vi "Conveyor_SendToServer.vi"(6 "Cluster":T1, 7 "Emergency":bool, 8 "State":string, 9 "RPM in":dbl(knob) scale=0.0..10.0, 10 "Speed in":i32(listbox), 11 "Temperature in":dbl(slide) scale=0.0..100.0) -> ()   [LabVIEW 2026]
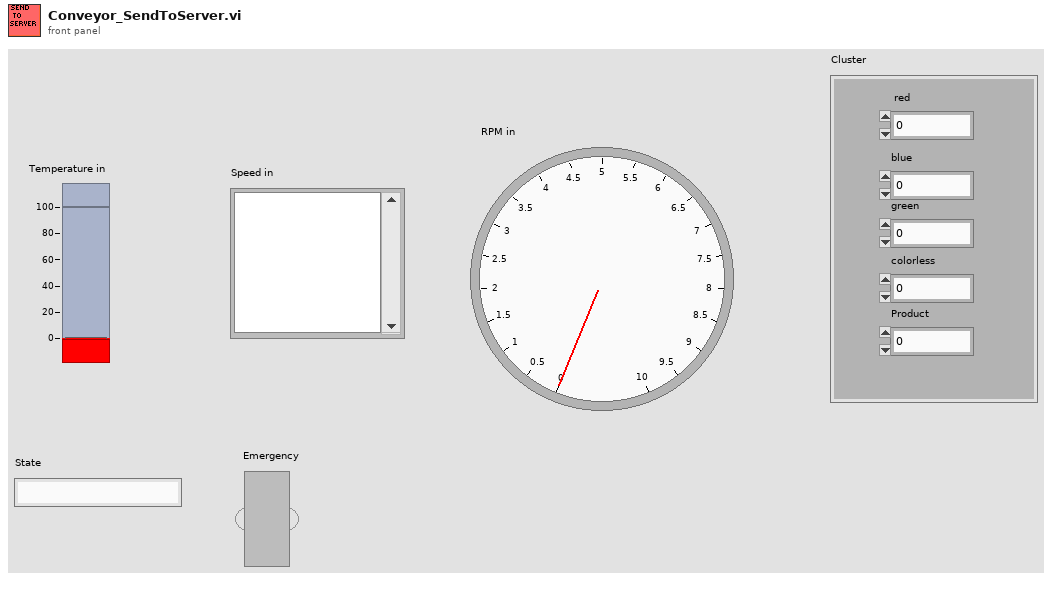
[diagram p1: front panel]
types:
  T1 = cluster{" red":i16, "blue":i16, "green":i16, "colorless":i16, "Product":i16}
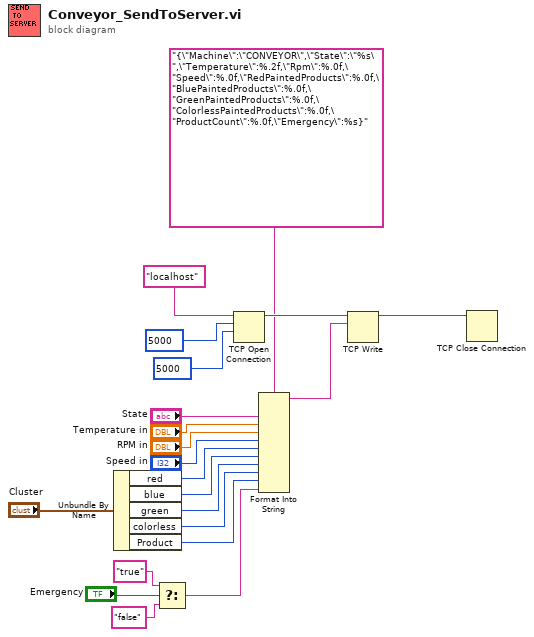
[diagram p0: block diagram]
diagram:
  n1 = Unbundle By Name("Cluster") -> ("red"=w5:i16, "blue"=w4:i16, "green"=w3:i16, "colorless"=w2:i16, "Product"=w1:i16)
  n2 = Select(t="true", s="Emergency", f="false") -> (s? t:f=w7:string)
  n3 = TCP Open Connection(address="localhost", remote port or service name=u16 5000, timeout ms (60000)=5000) -> (connection ID=w21:refnum<k5>)  [unwired: 2 in, 1 out]
  n4 = Format Into String(format string="{\"Machine\":\"CONVEYOR\",\"State\":\"%s\",\"Temperature\":%.2f,\"Rpm\":%.0f,\"Speed\":%.0f,\"RedPaintedProducts\":%.0f,\"BluePaintedProducts\":%.0f,\"GreenPaintedProducts\":%.0f,\"ColorlessPaintedProducts\":%.0f,\"ProductCount\":%.0f,\"Emergency\":%s}" ("initial string"), "State", "Temperature in", "RPM in", "Speed in", w5, w4, w3, w2, w1, w7) -> (resulting string=w11:string)  [unwired: 2 in, 1 out]
  n5 = TCP Write(connection ID=w21, data in=w11) -> (connection ID out=w20:refnum<k5>)  [unwired: 2 in, 2 out]
  n6 = TCP Close Connection(connection ID=w20) -> ()  [unwired: 2 in, 2 out]
